vi "Write Loop 1.vi"(7 "Enum - Menu":enum16{"INIT", "WRITE", "CLOSE"}(ring), 8 "error in (no error)":errorcluster) -> (0 "error out":errorcluster)   [LabVIEW 2025]
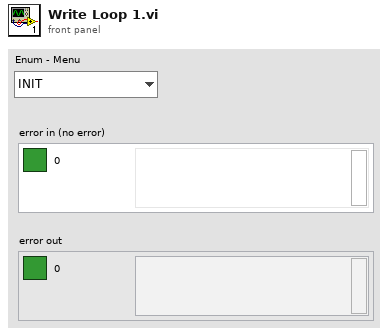
[diagram p1: front panel]
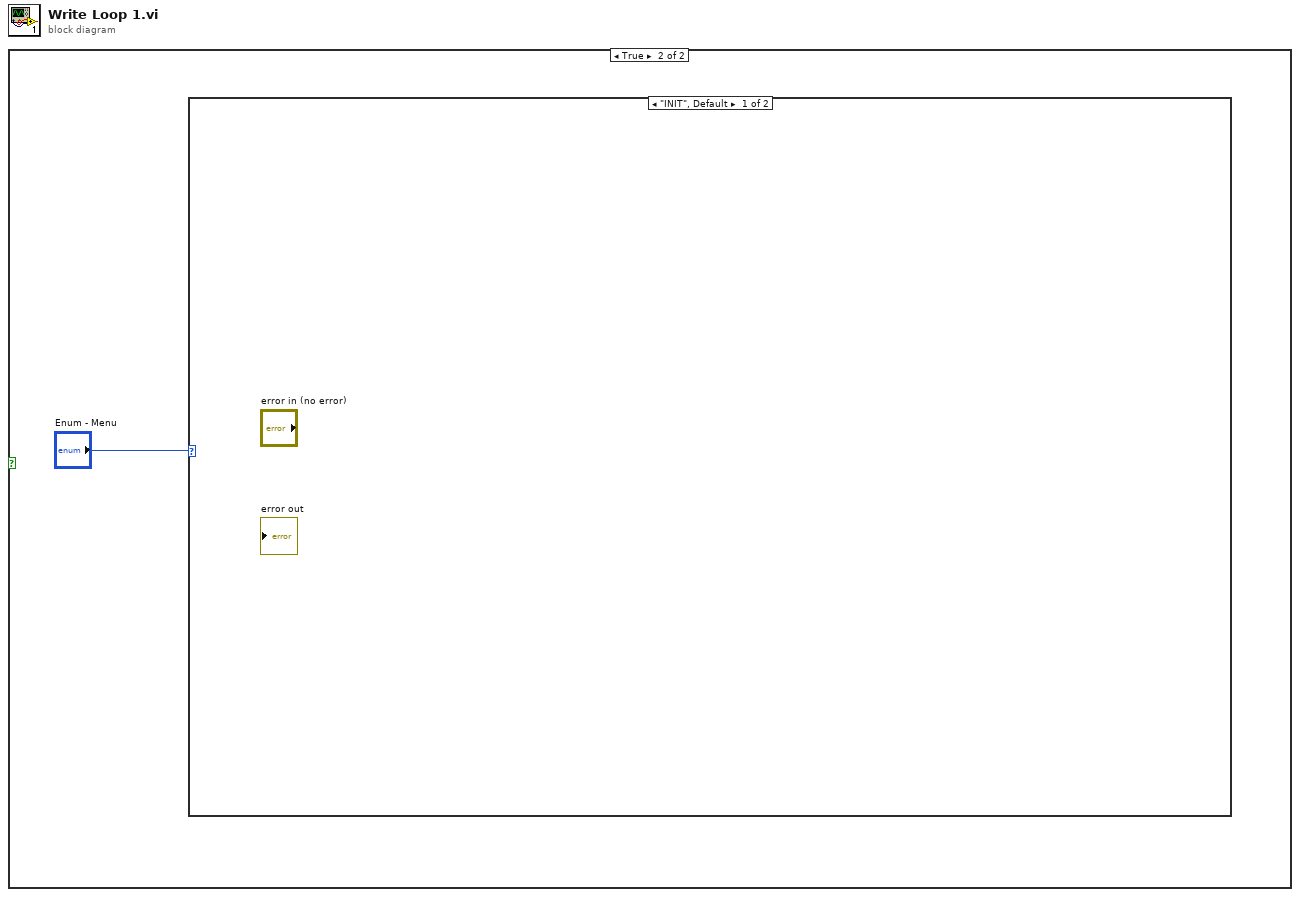
[diagram p0: block diagram]
diagram:
  n1 = case shown="True" {
    selector: _ -> [_ _]
    frame False {
    }
    frame True {
      n2 = case shown="\"INIT\", Default" "Enum - Menu" {
        frame "INIT", Default {
        }
        frame "WRITE" {
        }
      }
    }
  }
